vi "AWG_move.vi"(1 "Point":cluster{string, "data":u64, "data":dbl}, 2 "inst info":T1) -> (0 "error out":errorcluster)   [LabVIEW 2013]
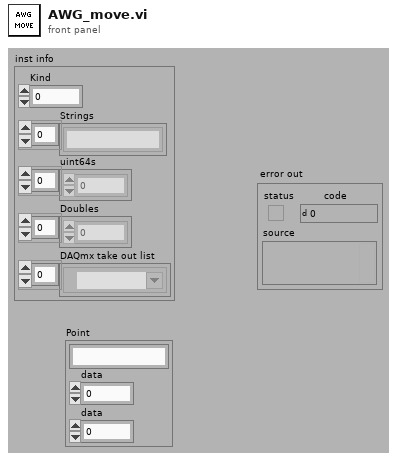
[diagram p1: front panel]
types:
  T1 = cluster{"Kind":u16, "Strings":string[], "uint64s":u64[], "Doubles":dbl[], "DAQmx take out list":refnum<k21>[]}
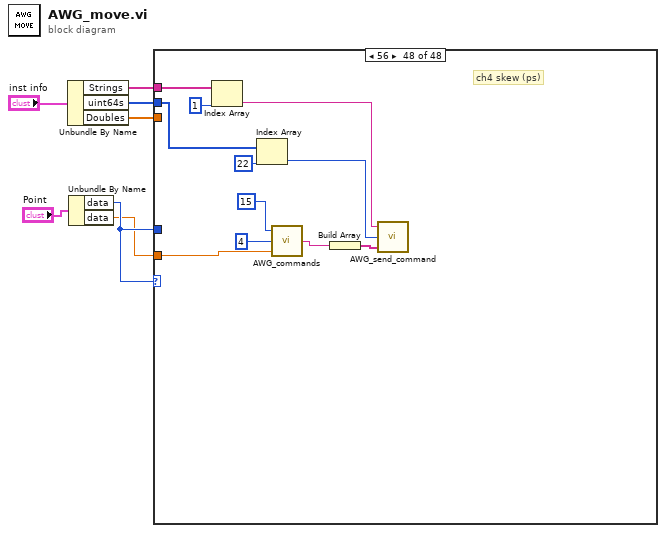
[diagram p0: block diagram]
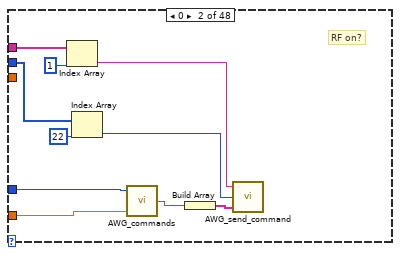
[diagram p3: hidden frame]
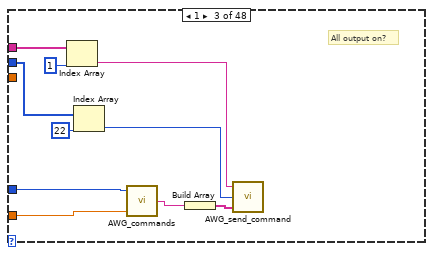
[diagram p4: hidden frame]
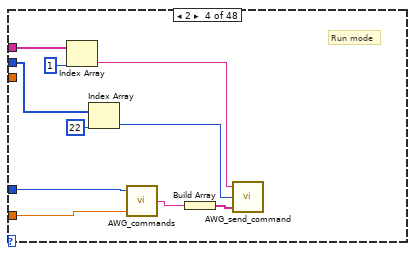
[diagram p5: hidden frame]
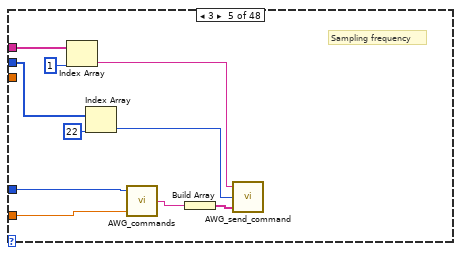
[diagram p6: hidden frame]
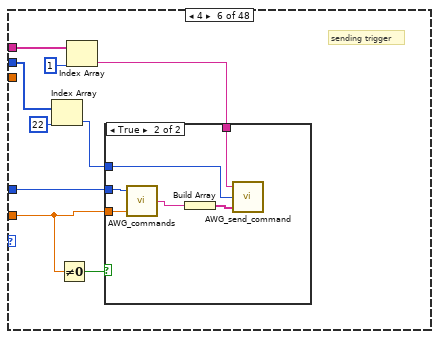
[diagram p7: hidden frame]
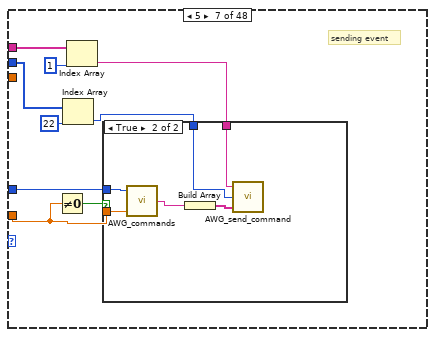
[diagram p9: hidden frame]
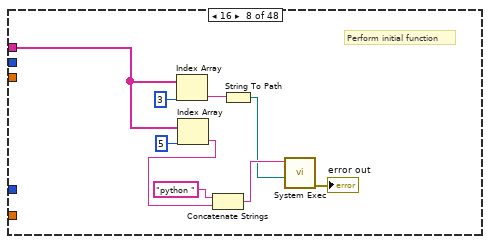
[diagram p11: hidden frame]
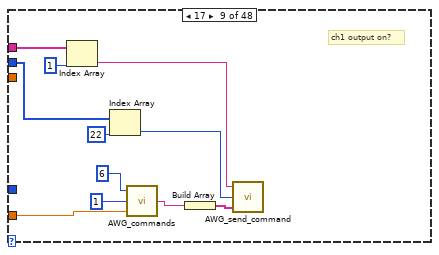
[diagram p12: hidden frame]
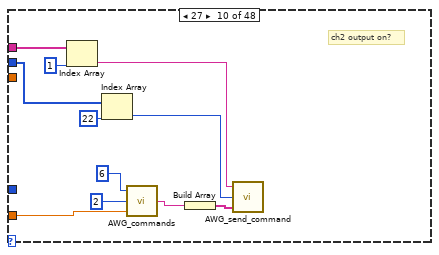
[diagram p13: hidden frame]
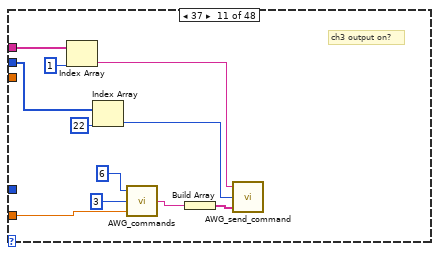
[diagram p14: hidden frame]
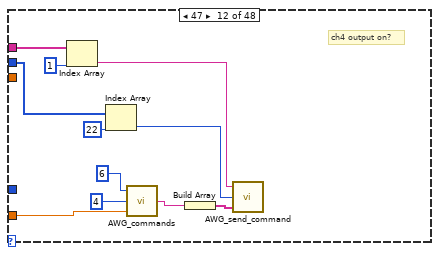
[diagram p15: hidden frame]
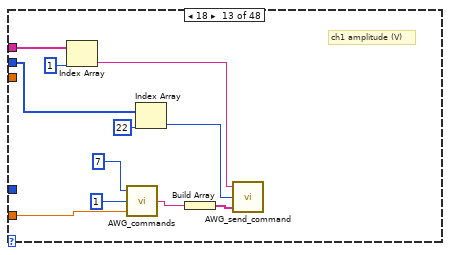
[diagram p16: hidden frame]
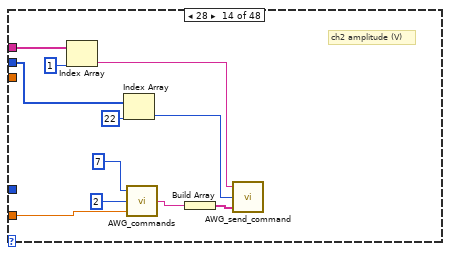
[diagram p17: hidden frame]
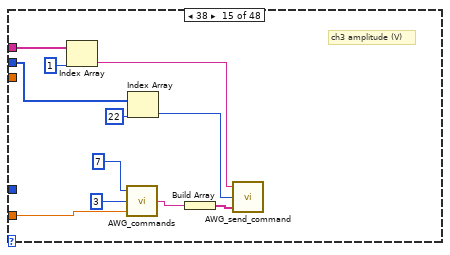
[diagram p18: hidden frame]
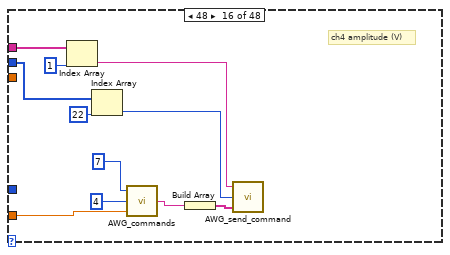
[diagram p19: hidden frame]
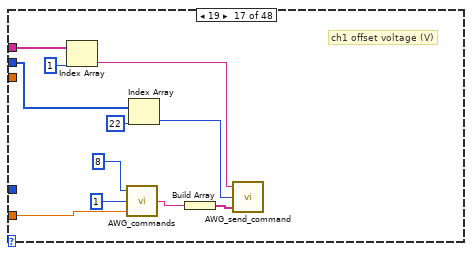
[diagram p20: hidden frame]
diagram:
  n1 = Unbundle By Name("inst info") -> ("Strings"=w5:string[], "uint64s"=w4:u64[], "Doubles"=w3:dbl[])
  n2 = Unbundle By Name("Point") -> ("data"=w7:u64, "data"=w6:dbl)
  n3 = case shown="56" w7 {
    tunnel: w7 -> [_ w17 w27 w37 w47 w56 w71 _ _ _ _ _ _ _ _ _ _ _ _ _ _ _ _ _ _ _ _ _ _ _ _ _ _ _ _ _ _ _ _ _ _ _ _ _ _ _ _ _]
    tunnel: w6 -> [_ w16 w26 w36 w46 w51 w66 _ w97 w108 w119 w130 w141 w152 w163 w174 w185 w196 w207 w218 w229 w240 w251 w262 w273 w284 w295 w306 w317 w328 w339 w350 w361 w372 w383 w394 w405 w416 w427 w438 w449 w460 w471 w482 w493 w504 w515 w526]
    tunnel: w5 -> [_ w15 w25 w35 w45 w55 w70 w84 w96 w107 w118 w129 w140 w151 w162 w173 w184 w195 w206 w217 w228 w239 w250 w261 w272 w283 w294 w305 w316 w327 w338 w349 w360 w371 w382 w393 w404 w415 w426 w437 w448 w459 w470 w481 w492 w503 w514 w525]
    tunnel: w4 -> [_ w9 w19 w29 w39 w49 w64 _ w88 w99 w110 w121 w132 w143 w154 w165 w176 w187 w198 w209 w220 w231 w242 w253 w264 w275 w286 w297 w308 w319 w330 w341 w352 w363 w374 w385 w396 w407 w418 w429 w440 w451 w462 w473 w484 w495 w506 w517]
    tunnel: w3 -> [_ _ _ _ _ _ _ _ _ _ _ _ _ _ _ _ _ _ _ _ _ _ _ _ _ _ _ _ _ _ _ _ _ _ _ _ _ _ _ _ _ _ _ _ _ _ _ _]
    frame 1000, Default {
    }
    frame 0 {
      # "RF on?"
      n4 = Index Array(array=w15, index=1) -> (element=w13:string)
      n5 = Index Array(array=w9, index=22) -> (element=w8:u64)
      n6 = call "AWG_commands.vi"("Value"=w16, "Commands"=w17) -> ("Comannd string"=w12:string)  [unwired: 1 in]
      n7 = Build Array(w12) -> (w11:string[])
      n8 = call "AWG_send_command.vi"("CMD list"=w11, "Port number"=w8, "IP Address"=w13) -> ()  [unwired: 1 in]
    }
    frame 1 {
      # "All output on?"
      n9 = Index Array(array=w25, index=1) -> (element=w23:string)
      n10 = Index Array(array=w19, index=22) -> (element=w18:u64)
      n11 = call "AWG_commands.vi"("Value"=w26, "Commands"=w27) -> ("Comannd string"=w22:string)  [unwired: 1 in]
      n12 = Build Array(w22) -> (w21:string[])
      n13 = call "AWG_send_command.vi"("CMD list"=w21, "Port number"=w18, "IP Address"=w23) -> ()  [unwired: 1 in]
    }
    frame 2 {
      # "Run mode"
      n14 = Index Array(array=w35, index=1) -> (element=w33:string)
      n15 = Index Array(array=w29, index=22) -> (element=w28:u64)
      n16 = call "AWG_commands.vi"("Value"=w36, "Commands"=w37) -> ("Comannd string"=w32:string)  [unwired: 1 in]
      n17 = Build Array(w32) -> (w31:string[])
      n18 = call "AWG_send_command.vi"("CMD list"=w31, "Port number"=w28, "IP Address"=w33) -> ()  [unwired: 1 in]
    }
    frame 3 {
      # "Sampling frequency"
      n19 = Index Array(array=w45, index=1) -> (element=w43:string)
      n20 = Index Array(array=w39, index=22) -> (element=w38:u64)
      n21 = call "AWG_commands.vi"("Value"=w46, "Commands"=w47) -> ("Comannd string"=w42:string)  [unwired: 1 in]
      n22 = Build Array(w42) -> (w41:string[])
      n23 = call "AWG_send_command.vi"("CMD list"=w41, "Port number"=w38, "IP Address"=w43) -> ()  [unwired: 1 in]
    }
    frame 4 {
      # "sending trigger"
      n24 = Index Array(array=w49, index=22) -> (element=w48:u64)
      n25 = Not Equal To 0?(x=w51) -> (x != 0?=w52:bool)
      n26 = Index Array(array=w55, index=1) -> (element=w53:string)
      n27 = case shown="True" w52 {
        tunnel: w56 -> [_ w62]
        tunnel: w51 -> [_ w61]
        tunnel: w53 -> [_ w60]
        tunnel: w48 -> [_ w57]
        frame False {
        }
        frame True {
          n28 = call "AWG_commands.vi"("Value"=w61, "Commands"=w62) -> ("Comannd string"=w59:string)  [unwired: 1 in]
          n29 = Build Array(w59) -> (w58:string[])
          n30 = call "AWG_send_command.vi"("CMD list"=w58, "Port number"=w57, "IP Address"=w60) -> ()  [unwired: 1 in]
        }
      }
    }
    frame 5 {
      # "sending event"
      n31 = Not Equal To 0?(x=w66) -> (x != 0?=w67:bool)
      n32 = Index Array(array=w64, index=22) -> (element=w63:u64)
      n33 = Index Array(array=w70, index=1) -> (element=w68:string)
      n34 = case shown="True" w67 {
        tunnel: w71 -> [_ w77]
        tunnel: w66 -> [_ w76]
        tunnel: w68 -> [_ w75]
        tunnel: w63 -> [_ w72]
        frame False {
        }
        frame True {
          n35 = call "AWG_commands.vi"("Value"=w76, "Commands"=w77) -> ("Comannd string"=w74:string)  [unwired: 1 in]
          n36 = Build Array(w74) -> (w73:string[])
          n37 = call "AWG_send_command.vi"("CMD list"=w73, "Port number"=w72, "IP Address"=w75) -> ()  [unwired: 1 in]
        }
      }
    }
    frame 16 {
      # "Perform initial function"
      n38 = Index Array(array=w84, index=3) -> (element=w83:string)
      n39 = Index Array(array=w84, index=5) -> (element=w79:string)
      n40 = Concatenate Strings("python ", w79) -> (w81:string)
      n41 = String To Path(string=w83) -> (path=w80:path)
      n42 = call <vilib>:"System Exec.vi"("working directory"=w80, "command line"=w81) -> ("error out"=→"error out":errorcluster)  [unwired: 6 in, 3 out]
    }
    frame 17 {
      # "ch1 output on?"
      n43 = Index Array(array=w96, index=1) -> (element=w94:string)
      n44 = Index Array(array=w88, index=22) -> (element=w87:u64)
      n45 = call "AWG_commands.vi"("Value"=w97, "Channel"=1, "Commands"=6) -> ("Comannd string"=w93:string)
      n46 = Build Array(w93) -> (w92:string[])
      n47 = call "AWG_send_command.vi"("CMD list"=w92, "Port number"=w87, "IP Address"=w94) -> ()  [unwired: 1 in]
    }
    frame 27 {
      # "ch2 output on?"
      n48 = Index Array(array=w107, index=1) -> (element=w105:string)
      n49 = Index Array(array=w99, index=22) -> (element=w98:u64)
      n50 = call "AWG_commands.vi"("Value"=w108, "Channel"=2, "Commands"=6) -> ("Comannd string"=w104:string)
      n51 = Build Array(w104) -> (w103:string[])
      n52 = call "AWG_send_command.vi"("CMD list"=w103, "Port number"=w98, "IP Address"=w105) -> ()  [unwired: 1 in]
    }
    frame 37 {
      # "ch3 output on?"
      n53 = Index Array(array=w118, index=1) -> (element=w116:string)
      n54 = Index Array(array=w110, index=22) -> (element=w109:u64)
      n55 = call "AWG_commands.vi"("Value"=w119, "Channel"=3, "Commands"=6) -> ("Comannd string"=w115:string)
      n56 = Build Array(w115) -> (w114:string[])
      n57 = call "AWG_send_command.vi"("CMD list"=w114, "Port number"=w109, "IP Address"=w116) -> ()  [unwired: 1 in]
    }
    frame 47 {
      # "ch4 output on?"
      n58 = Index Array(array=w129, index=1) -> (element=w127:string)
      n59 = Index Array(array=w121, index=22) -> (element=w120:u64)
      n60 = call "AWG_commands.vi"("Value"=w130, "Channel"=4, "Commands"=6) -> ("Comannd string"=w126:string)
      n61 = Build Array(w126) -> (w125:string[])
      n62 = call "AWG_send_command.vi"("CMD list"=w125, "Port number"=w120, "IP Address"=w127) -> ()  [unwired: 1 in]
    }
    frame 18 {
      # "ch1 amplitude (V)"
      n63 = Index Array(array=w140, index=1) -> (element=w138:string)
      n64 = call "AWG_commands.vi"("Value"=w141, "Channel"=1, "Commands"=7) -> ("Comannd string"=w137:string)
      n65 = Index Array(array=w132, index=22) -> (element=w131:u64)
      n66 = Build Array(w137) -> (w136:string[])
      n67 = call "AWG_send_command.vi"("CMD list"=w136, "Port number"=w131, "IP Address"=w138) -> ()  [unwired: 1 in]
    }
    frame 28 {
      # "ch2 amplitude (V)"
      n68 = Index Array(array=w151, index=1) -> (element=w149:string)
      n69 = Index Array(array=w143, index=22) -> (element=w142:u64)
      n70 = call "AWG_commands.vi"("Value"=w152, "Channel"=2, "Commands"=7) -> ("Comannd string"=w148:string)
      n71 = Build Array(w148) -> (w147:string[])
      n72 = call "AWG_send_command.vi"("CMD list"=w147, "Port number"=w142, "IP Address"=w149) -> ()  [unwired: 1 in]
    }
    frame 38 {
      # "ch3 amplitude (V)"
      n73 = Index Array(array=w162, index=1) -> (element=w160:string)
      n74 = call "AWG_commands.vi"("Value"=w163, "Channel"=3, "Commands"=7) -> ("Comannd string"=w159:string)
      n75 = Index Array(array=w154, index=22) -> (element=w153:u64)
      n76 = Build Array(w159) -> (w158:string[])
      n77 = call "AWG_send_command.vi"("CMD list"=w158, "Port number"=w153, "IP Address"=w160) -> ()  [unwired: 1 in]
    }
    frame 48 {
      # "ch4 amplitude (V)"
      n78 = Index Array(array=w173, index=1) -> (element=w171:string)
      n79 = Index Array(array=w165, index=22) -> (element=w164:u64)
      n80 = call "AWG_commands.vi"("Value"=w174, "Channel"=4, "Commands"=7) -> ("Comannd string"=w170:string)
      n81 = Build Array(w170) -> (w169:string[])
      n82 = call "AWG_send_command.vi"("CMD list"=w169, "Port number"=w164, "IP Address"=w171) -> ()  [unwired: 1 in]
    }
    frame 19 {
      # "ch1 offset voltage (V)"
      n83 = Index Array(array=w184, index=1) -> (element=w182:string)
      n84 = call "AWG_commands.vi"("Value"=w185, "Channel"=1, "Commands"=8) -> ("Comannd string"=w181:string)
      n85 = Index Array(array=w176, index=22) -> (element=w175:u64)
      n86 = Build Array(w181) -> (w180:string[])
      n87 = call "AWG_send_command.vi"("CMD list"=w180, "Port number"=w175, "IP Address"=w182) -> ()  [unwired: 1 in]
    }
    frame 29 {
      # "ch2 offset voltage (V)"
      n88 = Index Array(array=w195, index=1) -> (element=w193:string)
      n89 = call "AWG_commands.vi"("Value"=w196, "Channel"=2, "Commands"=8) -> ("Comannd string"=w192:string)
      n90 = Index Array(array=w187, index=22) -> (element=w186:u64)
      n91 = Build Array(w192) -> (w191:string[])
      n92 = call "AWG_send_command.vi"("CMD list"=w191, "Port number"=w186, "IP Address"=w193) -> ()  [unwired: 1 in]
    }
    frame 39 {
      # "ch3 offset voltage (V)"
      n93 = Index Array(array=w206, index=1) -> (element=w204:string)
      n94 = Index Array(array=w198, index=22) -> (element=w197:u64)
      n95 = call "AWG_commands.vi"("Value"=w207, "Channel"=3, "Commands"=8) -> ("Comannd string"=w203:string)
      n96 = Build Array(w203) -> (w202:string[])
      n97 = call "AWG_send_command.vi"("CMD list"=w202, "Port number"=w197, "IP Address"=w204) -> ()  [unwired: 1 in]
    }
    frame 49 {
      # "ch4 offset voltage (V)"
      n98 = Index Array(array=w217, index=1) -> (element=w215:string)
      n99 = call "AWG_commands.vi"("Value"=w218, "Channel"=4, "Commands"=8) -> ("Comannd string"=w214:string)
      n100 = Index Array(array=w209, index=22) -> (element=w208:u64)
      n101 = Build Array(w214) -> (w213:string[])
      n102 = call "AWG_send_command.vi"("CMD list"=w213, "Port number"=w208, "IP Address"=w215) -> ()  [unwired: 1 in]
    }
    frame 20 {
      # "ch1 marker1 high (V)"
      n103 = Index Array(array=w228, index=1) -> (element=w226:string)
      n104 = Index Array(array=w220, index=22) -> (element=w219:u64)
      n105 = call "AWG_commands.vi"("Value"=w229, "Channel"=1, "Commands"=9) -> ("Comannd string"=w225:string)
      n106 = Build Array(w225) -> (w224:string[])
      n107 = call "AWG_send_command.vi"("CMD list"=w224, "Port number"=w219, "IP Address"=w226) -> ()  [unwired: 1 in]
    }
    frame 30 {
      # "ch2 marker1 high (V)"
      n108 = Index Array(array=w239, index=1) -> (element=w237:string)
      n109 = Index Array(array=w231, index=22) -> (element=w230:u64)
      n110 = call "AWG_commands.vi"("Value"=w240, "Channel"=2, "Commands"=9) -> ("Comannd string"=w236:string)
      n111 = Build Array(w236) -> (w235:string[])
      n112 = call "AWG_send_command.vi"("CMD list"=w235, "Port number"=w230, "IP Address"=w237) -> ()  [unwired: 1 in]
    }
    frame 40 {
      # "ch3 marker1 high (V)"
      n113 = Index Array(array=w250, index=1) -> (element=w248:string)
      n114 = Index Array(array=w242, index=22) -> (element=w241:u64)
      n115 = call "AWG_commands.vi"("Value"=w251, "Channel"=3, "Commands"=9) -> ("Comannd string"=w247:string)
      n116 = Build Array(w247) -> (w246:string[])
      n117 = call "AWG_send_command.vi"("CMD list"=w246, "Port number"=w241, "IP Address"=w248) -> ()  [unwired: 1 in]
    }
    frame 50 {
      # "ch4 marker1 high (V)"
      n118 = Index Array(array=w261, index=1) -> (element=w259:string)
      n119 = call "AWG_commands.vi"("Value"=w262, "Channel"=4, "Commands"=9) -> ("Comannd string"=w258:string)
      n120 = Index Array(array=w253, index=22) -> (element=w252:u64)
      n121 = Build Array(w258) -> (w257:string[])
      n122 = call "AWG_send_command.vi"("CMD list"=w257, "Port number"=w252, "IP Address"=w259) -> ()  [unwired: 1 in]
    }
    frame 21 {
      # "ch1 marker1 low (V)"
      n123 = Index Array(array=w272, index=1) -> (element=w270:string)
      n124 = Index Array(array=w264, index=22) -> (element=w263:u64)
      n125 = call "AWG_commands.vi"("Value"=w273, "Channel"=1, "Commands"=10) -> ("Comannd string"=w269:string)
      n126 = Build Array(w269) -> (w268:string[])
      n127 = call "AWG_send_command.vi"("CMD list"=w268, "Port number"=w263, "IP Address"=w270) -> ()  [unwired: 1 in]
    }
    frame 31 {
      # "ch2 marker1 low (V)"
      n128 = Index Array(array=w283, index=1) -> (element=w281:string)
      n129 = Index Array(array=w275, index=22) -> (element=w274:u64)
      n130 = call "AWG_commands.vi"("Value"=w284, "Channel"=2, "Commands"=10) -> ("Comannd string"=w280:string)
      n131 = Build Array(w280) -> (w279:string[])
      n132 = call "AWG_send_command.vi"("CMD list"=w279, "Port number"=w274, "IP Address"=w281) -> ()  [unwired: 1 in]
    }
    frame 41 {
      # "ch3 marker1 low (V)"
      n133 = Index Array(array=w294, index=1) -> (element=w292:string)
      n134 = Index Array(array=w286, index=22) -> (element=w285:u64)
      n135 = call "AWG_commands.vi"("Value"=w295, "Channel"=3, "Commands"=10) -> ("Comannd string"=w291:string)
      n136 = Build Array(w291) -> (w290:string[])
      n137 = call "AWG_send_command.vi"("CMD list"=w290, "Port number"=w285, "IP Address"=w292) -> ()  [unwired: 1 in]
    }
    frame 51 {
      # "ch4 marker1 low (V)"
      n138 = Index Array(array=w305, index=1) -> (element=w303:string)
      n139 = Index Array(array=w297, index=22) -> (element=w296:u64)
      n140 = call "AWG_commands.vi"("Value"=w306, "Channel"=4, "Commands"=10) -> ("Comannd string"=w302:string)
      n141 = Build Array(w302) -> (w301:string[])
      n142 = call "AWG_send_command.vi"("CMD list"=w301, "Port number"=w296, "IP Address"=w303) -> ()  [unwired: 1 in]
    }
    frame 22 {
      # "ch1 marker1 delay (ps)"
      n143 = Index Array(array=w316, index=1) -> (element=w314:string)
      n144 = Index Array(array=w308, index=22) -> (element=w307:u64)
      n145 = call "AWG_commands.vi"("Value"=w317, "Channel"=1, "Commands"=11) -> ("Comannd string"=w313:string)
      n146 = Build Array(w313) -> (w312:string[])
      n147 = call "AWG_send_command.vi"("CMD list"=w312, "Port number"=w307, "IP Address"=w314) -> ()  [unwired: 1 in]
    }
    frame 32 {
      # "ch2 marker1 delay (ps)"
      n148 = Index Array(array=w327, index=1) -> (element=w325:string)
      n149 = Index Array(array=w319, index=22) -> (element=w318:u64)
      n150 = call "AWG_commands.vi"("Value"=w328, "Channel"=2, "Commands"=11) -> ("Comannd string"=w324:string)
      n151 = Build Array(w324) -> (w323:string[])
      n152 = call "AWG_send_command.vi"("CMD list"=w323, "Port number"=w318, "IP Address"=w325) -> ()  [unwired: 1 in]
    }
    frame 42 {
      # "ch3 marker1 delay (ps)"
      n153 = Index Array(array=w338, index=1) -> (element=w336:string)
      n154 = Index Array(array=w330, index=22) -> (element=w329:u64)
      n155 = call "AWG_commands.vi"("Value"=w339, "Channel"=3, "Commands"=11) -> ("Comannd string"=w335:string)
      n156 = Build Array(w335) -> (w334:string[])
      n157 = call "AWG_send_command.vi"("CMD list"=w334, "Port number"=w329, "IP Address"=w336) -> ()  [unwired: 1 in]
    }
    frame 52 {
      # "ch4 marker1 delay (ps)"
      n158 = Index Array(array=w349, index=1) -> (element=w347:string)
      n159 = Index Array(array=w341, index=22) -> (element=w340:u64)
      n160 = call "AWG_commands.vi"("Value"=w350, "Channel"=4, "Commands"=11) -> ("Comannd string"=w346:string)
      n161 = Build Array(w346) -> (w345:string[])
      n162 = call "AWG_send_command.vi"("CMD list"=w345, "Port number"=w340, "IP Address"=w347) -> ()  [unwired: 1 in]
    }
    frame 23 {
      # "ch1 marker2 high (V)"
      n163 = Index Array(array=w360, index=1) -> (element=w358:string)
      n164 = Index Array(array=w352, index=22) -> (element=w351:u64)
      n165 = call "AWG_commands.vi"("Value"=w361, "Channel"=1, "Commands"=12) -> ("Comannd string"=w357:string)
      n166 = Build Array(w357) -> (w356:string[])
      n167 = call "AWG_send_command.vi"("CMD list"=w356, "Port number"=w351, "IP Address"=w358) -> ()  [unwired: 1 in]
    }
    frame 33 {
      # "ch2 marker2 high (V)"
      n168 = Index Array(array=w371, index=1) -> (element=w369:string)
      n169 = Index Array(array=w363, index=22) -> (element=w362:u64)
      n170 = call "AWG_commands.vi"("Value"=w372, "Channel"=2, "Commands"=12) -> ("Comannd string"=w368:string)
      n171 = Build Array(w368) -> (w367:string[])
      n172 = call "AWG_send_command.vi"("CMD list"=w367, "Port number"=w362, "IP Address"=w369) -> ()  [unwired: 1 in]
    }
    frame 43 {
      # "ch3 marker2 high (V)"
      n173 = Index Array(array=w382, index=1) -> (element=w380:string)
      n174 = call "AWG_commands.vi"("Value"=w383, "Channel"=3, "Commands"=12) -> ("Comannd string"=w379:string)
      n175 = Index Array(array=w374, index=22) -> (element=w373:u64)
      n176 = Build Array(w379) -> (w378:string[])
      n177 = call "AWG_send_command.vi"("CMD list"=w378, "Port number"=w373, "IP Address"=w380) -> ()  [unwired: 1 in]
    }
    frame 53 {
      # "ch4 marker2 high (V)"
      n178 = Index Array(array=w393, index=1) -> (element=w391:string)
      n179 = Index Array(array=w385, index=22) -> (element=w384:u64)
      n180 = call "AWG_commands.vi"("Value"=w394, "Channel"=4, "Commands"=12) -> ("Comannd string"=w390:string)
      n181 = Build Array(w390) -> (w389:string[])
      n182 = call "AWG_send_command.vi"("CMD list"=w389, "Port number"=w384, "IP Address"=w391) -> ()  [unwired: 1 in]
    }
    frame 24 {
      # "ch1 marker2 low (V)"
      n183 = Index Array(array=w404, index=1) -> (element=w402:string)
      n184 = Index Array(array=w396, index=22) -> (element=w395:u64)
      n185 = call "AWG_commands.vi"("Value"=w405, "Channel"=1, "Commands"=13) -> ("Comannd string"=w401:string)
      n186 = Build Array(w401) -> (w400:string[])
      n187 = call "AWG_send_command.vi"("CMD list"=w400, "Port number"=w395, "IP Address"=w402) -> ()  [unwired: 1 in]
    }
    frame 34 {
      # "ch2 marker2 low (V)"
      n188 = Index Array(array=w415, index=1) -> (element=w413:string)
      n189 = Index Array(array=w407, index=22) -> (element=w406:u64)
      n190 = call "AWG_commands.vi"("Value"=w416, "Channel"=2, "Commands"=13) -> ("Comannd string"=w412:string)
      n191 = Build Array(w412) -> (w411:string[])
      n192 = call "AWG_send_command.vi"("CMD list"=w411, "Port number"=w406, "IP Address"=w413) -> ()  [unwired: 1 in]
    }
    frame 44 {
      # "ch3 marker2 low (V)"
      n193 = Index Array(array=w426, index=1) -> (element=w424:string)
      n194 = Index Array(array=w418, index=22) -> (element=w417:u64)
      n195 = call "AWG_commands.vi"("Value"=w427, "Channel"=3, "Commands"=13) -> ("Comannd string"=w423:string)
      n196 = Build Array(w423) -> (w422:string[])
      n197 = call "AWG_send_command.vi"("CMD list"=w422, "Port number"=w417, "IP Address"=w424) -> ()  [unwired: 1 in]
    }
    frame 54 {
      # "ch4 marker2 low (V)"
      n198 = Index Array(array=w437, index=1) -> (element=w435:string)
      n199 = Index Array(array=w429, index=22) -> (element=w428:u64)
      n200 = call "AWG_commands.vi"("Value"=w438, "Channel"=4, "Commands"=13) -> ("Comannd string"=w434:string)
      n201 = Build Array(w434) -> (w433:string[])
      n202 = call "AWG_send_command.vi"("CMD list"=w433, "Port number"=w428, "IP Address"=w435) -> ()  [unwired: 1 in]
    }
    frame 25 {
      # "ch1 marker2 delay (ps)"
      n203 = Index Array(array=w448, index=1) -> (element=w446:string)
      n204 = Index Array(array=w440, index=22) -> (element=w439:u64)
      n205 = call "AWG_commands.vi"("Value"=w449, "Channel"=1, "Commands"=14) -> ("Comannd string"=w445:string)
      n206 = Build Array(w445) -> (w444:string[])
      n207 = call "AWG_send_command.vi"("CMD list"=w444, "Port number"=w439, "IP Address"=w446) -> ()  [unwired: 1 in]
    }
    frame 35 {
      # "ch2 marker2 delay (ps)"
      n208 = Index Array(array=w459, index=1) -> (element=w457:string)
      n209 = Index Array(array=w451, index=22) -> (element=w450:u64)
      n210 = call "AWG_commands.vi"("Value"=w460, "Channel"=2, "Commands"=14) -> ("Comannd string"=w456:string)
      n211 = Build Array(w456) -> (w455:string[])
      n212 = call "AWG_send_command.vi"("CMD list"=w455, "Port number"=w450, "IP Address"=w457) -> ()  [unwired: 1 in]
    }
    frame 45 {
      # "ch3 marker2 delay (ps)"
      n213 = Index Array(array=w470, index=1) -> (element=w468:string)
      n214 = Index Array(array=w462, index=22) -> (element=w461:u64)
      n215 = call "AWG_commands.vi"("Value"=w471, "Channel"=3, "Commands"=14) -> ("Comannd string"=w467:string)
      n216 = Build Array(w467) -> (w466:string[])
      n217 = call "AWG_send_command.vi"("CMD list"=w466, "Port number"=w461, "IP Address"=w468) -> ()  [unwired: 1 in]
    }
    frame 55 {
      # "ch4 marker2 delay (ps)"
      n218 = Index Array(array=w481, index=1) -> (element=w479:string)
      n219 = call "AWG_commands.vi"("Value"=w482, "Channel"=4, "Commands"=14) -> ("Comannd string"=w478:string)
      n220 = Index Array(array=w473, index=22) -> (element=w472:u64)
      n221 = Build Array(w478) -> (w477:string[])
      n222 = call "AWG_send_command.vi"("CMD list"=w477, "Port number"=w472, "IP Address"=w479) -> ()  [unwired: 1 in]
    }
    frame 26 {
      # "ch1 skew (ps)"
      n223 = Index Array(array=w492, index=1) -> (element=w490:string)
      n224 = Index Array(array=w484, index=22) -> (element=w483:u64)
      n225 = call "AWG_commands.vi"("Value"=w493, "Channel"=1, "Commands"=15) -> ("Comannd string"=w489:string)
      n226 = Build Array(w489) -> (w488:string[])
      n227 = call "AWG_send_command.vi"("CMD list"=w488, "Port number"=w483, "IP Address"=w490) -> ()  [unwired: 1 in]
    }
    frame 36 {
      # "ch2 skew (ps)"
      n228 = Index Array(array=w503, index=1) -> (element=w501:string)
      n229 = call "AWG_commands.vi"("Value"=w504, "Channel"=2, "Commands"=15) -> ("Comannd string"=w500:string)
      n230 = Index Array(array=w495, index=22) -> (element=w494:u64)
      n231 = Build Array(w500) -> (w499:string[])
      n232 = call "AWG_send_command.vi"("CMD list"=w499, "Port number"=w494, "IP Address"=w501) -> ()  [unwired: 1 in]
    }
    frame 46 {
      # "ch3 skew (ps)"
      n233 = Index Array(array=w514, index=1) -> (element=w512:string)
      n234 = Index Array(array=w506, index=22) -> (element=w505:u64)
      n235 = call "AWG_commands.vi"("Value"=w515, "Channel"=3, "Commands"=15) -> ("Comannd string"=w511:string)
      n236 = Build Array(w511) -> (w510:string[])
      n237 = call "AWG_send_command.vi"("CMD list"=w510, "Port number"=w505, "IP Address"=w512) -> ()  [unwired: 1 in]
    }
    frame 56 {
      # "ch4 skew (ps)"
      n238 = Index Array(array=w525, index=1) -> (element=w523:string)
      n239 = Index Array(array=w517, index=22) -> (element=w516:u64)
      n240 = call "AWG_commands.vi"("Value"=w526, "Channel"=4, "Commands"=15) -> ("Comannd string"=w522:string)
      n241 = Build Array(w522) -> (w521:string[])
      n242 = call "AWG_send_command.vi"("CMD list"=w521, "Port number"=w516, "IP Address"=w523) -> ()  [unwired: 1 in]
    }
  }
